vi "Get SGL Array from Image.vi"(8 "error in (no error)":errorcluster, 9 "Image Array in (Empty)":dbl[][](array[numeric]), 11 "Image Refnum in":T1) -> (0 "error out":errorcluster, 1 "Image Array out":dbl[][](array[numeric]), 3 "Image Refnum dup":T1)   [LabVIEW 2021, in "Image.lvlib"]
doc: "Extract SGL Array from SGL image.\nFor other image types, the returned array is empty.\nIf there is an error before this VI executes, the input array (default: empty) is returned."
uses:
  <vilib>/vision/Image Controls.llb/IMAQ Image.ctl
  Image.lvlib
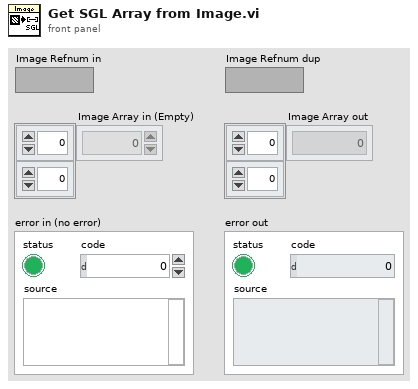
[diagram p1: front panel]
types:
  T1 = typedef "IMAQ Image.ctl" = refnum<image>
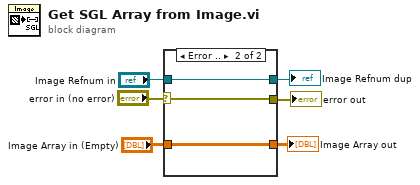
[diagram p0: block diagram]
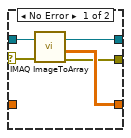
[diagram p2: hidden frame]
diagram:
  n1 = case shown="Error .." "error in (no error)" {
    selector: "error in (no error)" -> [w10 w12]
    tunnel: "Image Refnum in" -> [w7 w11]
    tunnel: [w9 w13] -> w4
    tunnel: [w8 w12] -> w3
    tunnel: "Image Array in (Empty)" -> [_ w13]
    tunnel: [w7 w11] -> w1
    frame No Error {
      n2 = call "IMAQ ImageToArray"("error in (no error)"=w10, "Image"=w7) -> ("Image Pixels (Float)"=w9:sgl[][], "error out"=w8:errorcluster)  [unwired: 2 in, 3 out]
    }
    frame Error {
    }
  }
  "error out" <- w3
  "Image Array out" <- w4
  "Image Refnum dup" <- w1
